vi "main.vi"() -> ()   [LabVIEW 2015]
uses:
  status.ctl
  states.ctl
  <vilib>/Analysis/1siggen.llb/Riffle Array (I32).vi
  <vilib>/Analysis/NI_AALBase.lvlib
panel:
  out "Session Info":T1
  out "Status":T2
  in  "Number of trials 2":u16=100
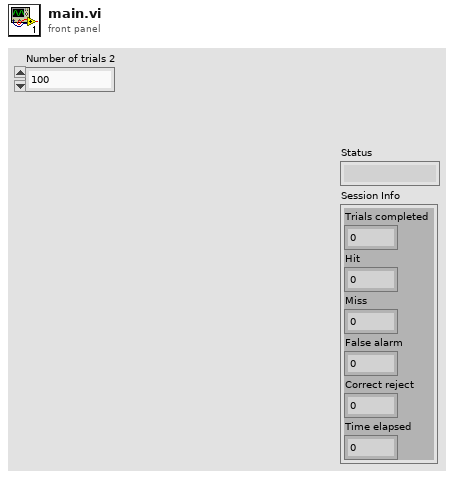
[diagram p1: front panel]
types:
  T1 = cluster{"Trials completed":i32, "Hit":i32, "Miss":i32, "False alarm":i32, "Correct reject":i32, "Time elapsed":i32}
  T2 = typedef "status.ctl" = string
  T3 = typedef "states.ctl" = enum16{"Initialization", "ITI", "Trial +", "Trial -", "Stop", "Error"}
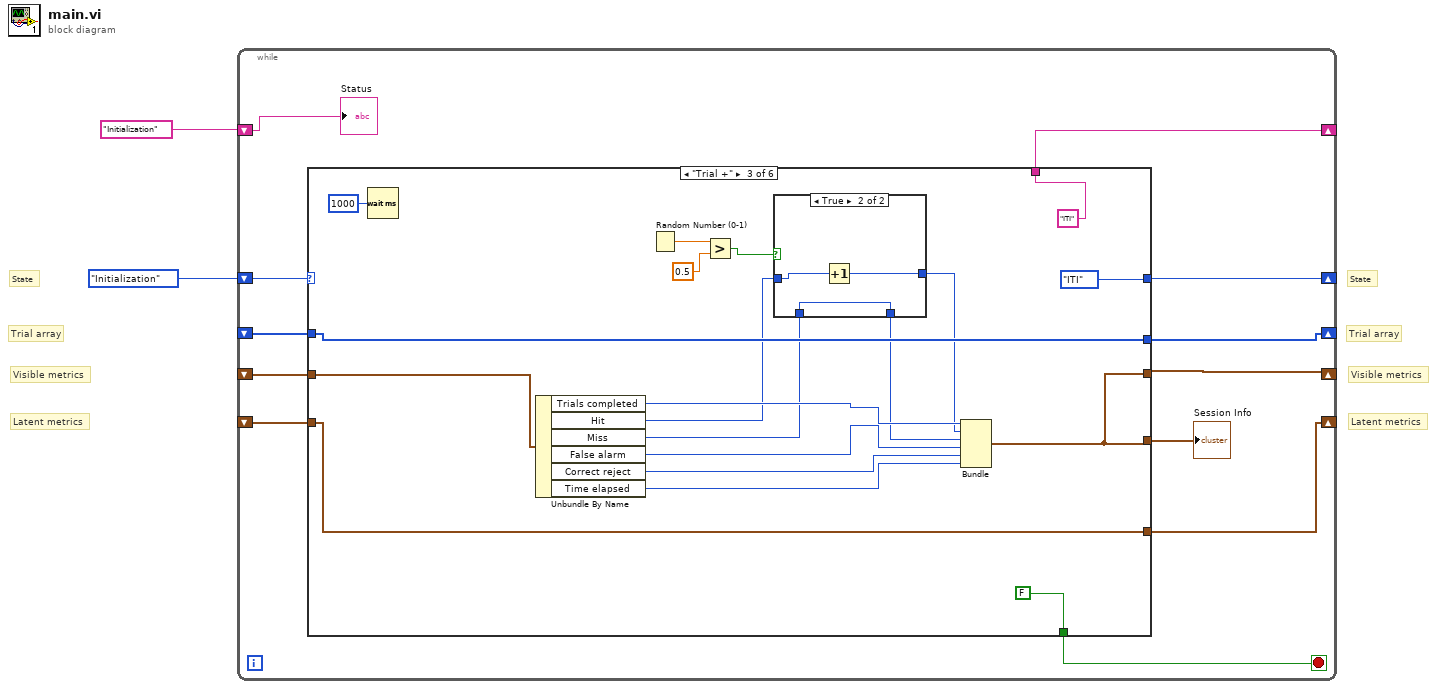
[diagram p0: block diagram]
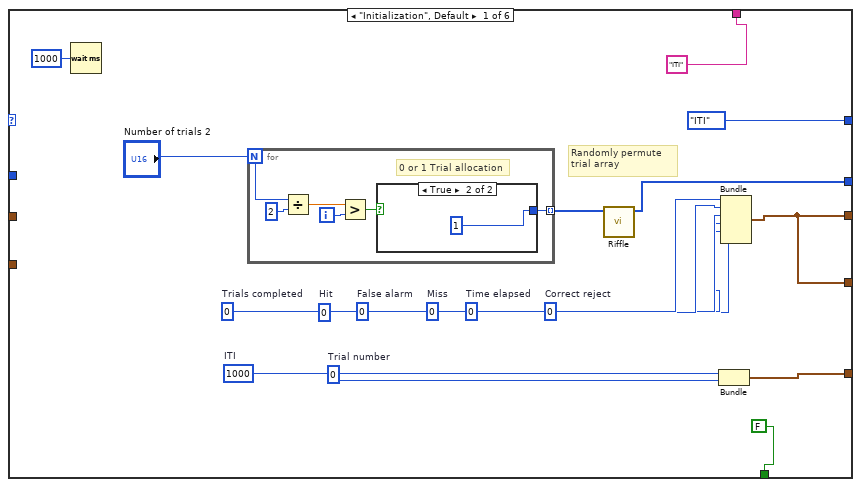
[diagram p2: hidden frame]
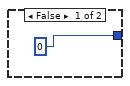
[diagram p3: hidden frame]
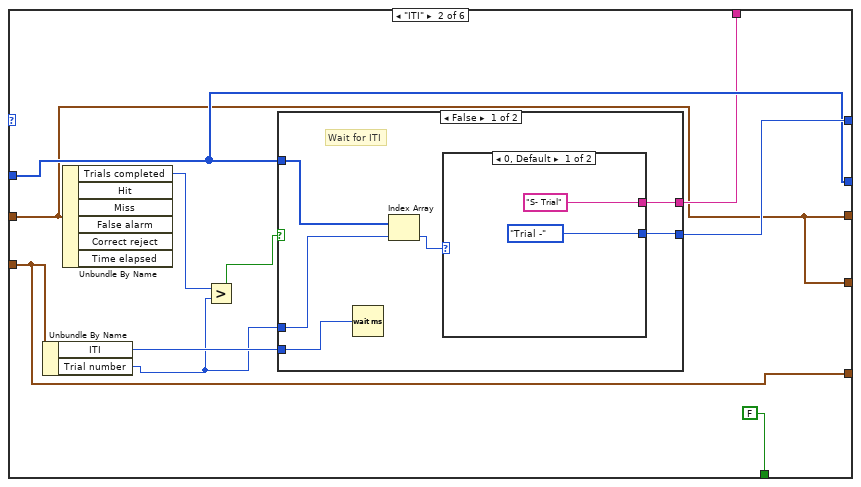
[diagram p4: hidden frame]
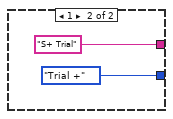
[diagram p5: hidden frame]
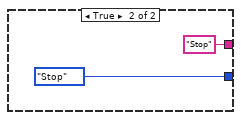
[diagram p6: hidden frame]
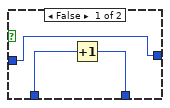
[diagram p7: hidden frame]
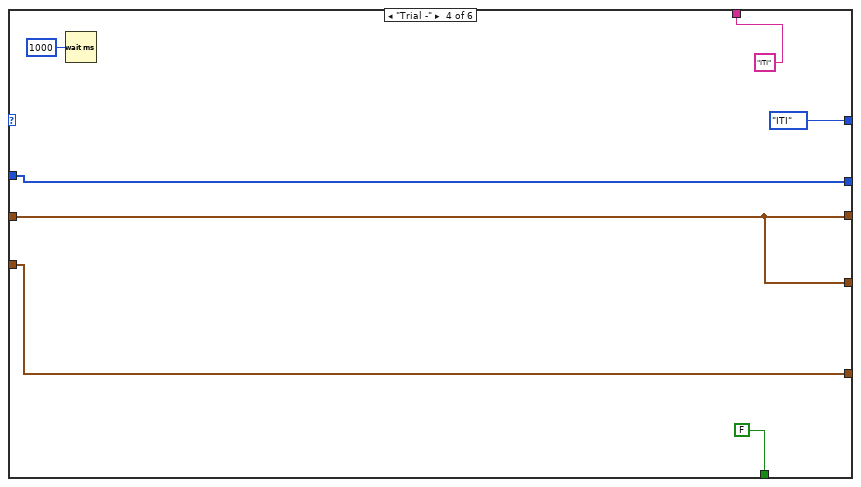
[diagram p8: hidden frame]
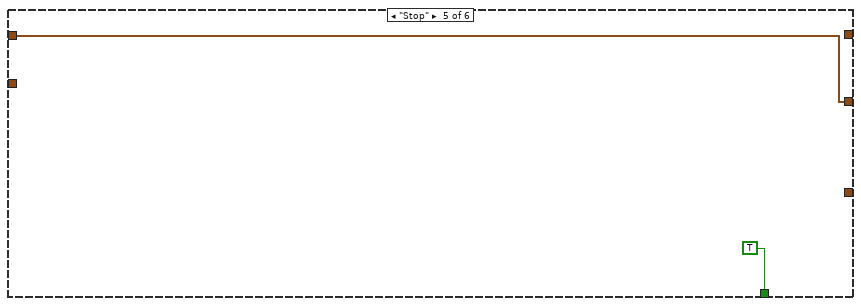
[diagram p9: hidden frame]
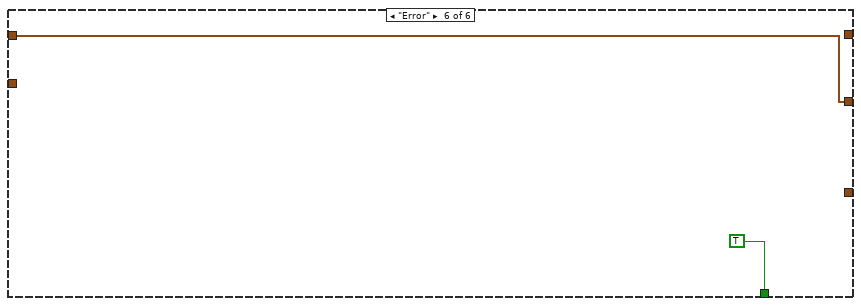
[diagram p10: hidden frame]
diagram:
  # "Latent metrics"
  # "Visible metrics"
  # "Trial array"
  # "State"
  # "Latent metrics"
  # "Visible metrics"
  # "Trial array"
  # "State"
  n1 = while {
    shift-right: [w13] -> _
    shift-left: states."Initialization" -> [w14]
    shift-right: [w12] -> _
    shift-left: _ -> [w8]
    shift-right: [w11] -> _
    shift-left: _ -> [w7]
    shift-right: [w10] -> _
    shift-left: _ -> [w9]
    shift-right: [w5] -> _
    shift-left: "Initialization" -> [w4]
    stop <- w6 stop-if-true
    n2 = case shown="\"Trial +\"" w14 {
      tunnel: [states."ITI" w47 states."ITI" states."ITI" _ _] -> w13
      tunnel: [w15 w40 w62 w87 _ _] -> w12
      tunnel: [w22 w44 w78 w91 _ _] -> w11
      tunnel: [w20 w43 w77 w90 _ _] -> w10
      tunnel: w9 -> [_ w43 w77 w90 _ _]
      tunnel: w8 -> [_ w40 w63 w87 w94 w96]
      tunnel: w7 -> [_ w44 w78 w91 _ _]
      tunnel: [FALSE FALSE FALSE FALSE TRUE TRUE] -> w6
      tunnel: ["ITI" w41 "ITI" "ITI" _ _] -> w5
      tunnel: [w15 w40 w62 w87 w94 w96] -> w3
      frame "Initialization", Default {
        w19 = 0  # Trial number
        w21 = 1000  # ITI
        w23 = 0  # Time elapsed
        w25 = 0  # False alarm
        w24 = 0  # Correct reject
        w26 = 0  # Miss
        w27 = 0  # Hit
        w28 = 0  # Trials completed
        # "Randomly permute \ntrial array"
        n3 = Wait (ms)(milliseconds to wait=u32 1000) -> ()  [unwired: 1 out]
        n4 = for {
          N: "Number of trials 2" -> [w36]
          tunnel: [w32] -> w30 mode=indexing
          i -> [w37]
          # "0 or 1 Trial allocation"
          n5 = Divide(x=w36, y=2) -> (x/y=w34:dbl)
          n6 = Greater?(x=w34, y=w37) -> (0:w33:bool)
          n7 = case shown="True" w33 {
            tunnel: [0 1] -> w32
            frame False {
            }
            frame True {
            }
          }
        }
        n8 = call-poly <vilib>:"Riffle.vi"("X"=w30) -> ("Riffled {X}"=w22:i32[])  [unwired: 8 in, 2 out]
        n9 = Bundle("ITI"=w21, "Trial number"=w19) -> (w20:cluster{"ITI":i32, "Trial number":i32})  [unwired: 1 in]
        n10 = Bundle("Trials completed"=w28, "Hit"=w27, "Miss"=w26, "False alarm"=w25, "Correct reject"=w24, "Time elapsed"=w23) -> (w15:T1)  [unwired: 1 in]
      }
      frame "ITI" {
        n11 = Unbundle By Name(w43) -> ("ITI"=w46:i32, "Trial number"=w45:i32)
        n12 = Unbundle By Name(w40) -> ("Trials completed"=w48:i32)  [unwired: 5 out]
        n13 = Greater?(x=w48, y=w45) -> (0:w49:bool)
        n14 = case shown="False" w49 {
          tunnel: [w51 states."Stop"] -> w47
          tunnel: w46 -> [w55 _]
          tunnel: w44 -> [w54 _]
          tunnel: w45 -> [w53 _]
          tunnel: [w50 "Stop"] -> w41
          frame False {
            # "Wait for ITI"
            n15 = Wait (ms)(milliseconds to wait=w55) -> ()  [unwired: 1 out]
            n16 = Index Array(array=w54, index=w53) -> (element=w52:i32)
            n17 = case shown="0, Default" w52 {
              tunnel: [states."Trial -" states."Trial +"] -> w51
              tunnel: ["S- Trial" "S+ Trial"] -> w50
              frame 0, Default {
              }
              frame 1 {
              }
            }
          }
          frame True {
          }
        }
      }
      frame "Trial +" {
        n18 = Wait (ms)(milliseconds to wait=u32 1000) -> ()  [unwired: 1 out]
        n19 = Unbundle By Name(w63) -> ("Trials completed"=w72:i32, "Hit"=w67:i32, "Miss"=w66:i32, "False alarm"=w71:i32, "Correct reject"=w70:i32, "Time elapsed"=w69:i32)
        n20 = Random Number (0-1)() -> (number: 0 to 1=w74:dbl)
        n21 = Greater?(x=w74, y=0.5) -> (0:w68:bool)
        n22 = case shown="True" w68 {
          tunnel: w67 -> [w81 w86]
          tunnel: w66 -> [w83 w85]
          tunnel: [w81 w84] -> w65
          tunnel: [w82 w85] -> w64
          frame False {
            n23 = Increment(x=w83) -> (x+1=w82:i32)
          }
          frame True {
            n24 = Increment(x=w86) -> (x+1=w84:i32)
          }
        }
        n25 = Bundle("Trials completed"=w72, "Hit"=w65, "Miss"=w64, "False alarm"=w71, "Correct reject"=w70, "Time elapsed"=w69) -> (w62:T1)  [unwired: 1 in]
      }
      frame "Trial -" {
        n26 = Wait (ms)(milliseconds to wait=u32 1000) -> ()  [unwired: 1 out]
      }
      frame "Stop" {
      }
      frame "Error" {
      }
    }
    "Session Info" <- w3
    "Status" <- w4
  }
